vi "SW_Make_Track_overlay.vi"(4 "Pen properties":T1, 5 "Full track array":T2(array[cluster]), 6 "Full trace color":u32(colorbox)=16711680, 7 "Picture in":picture) -> (1 "Picture out":picture)   [LabVIEW 2016]
panel:
  in  "Input colors array":u32[](array[colorbox])=[255, 65535, 6618880, 16776960, 16744448, 16711680]
  out "Colors array":u32[](array[colorbox])
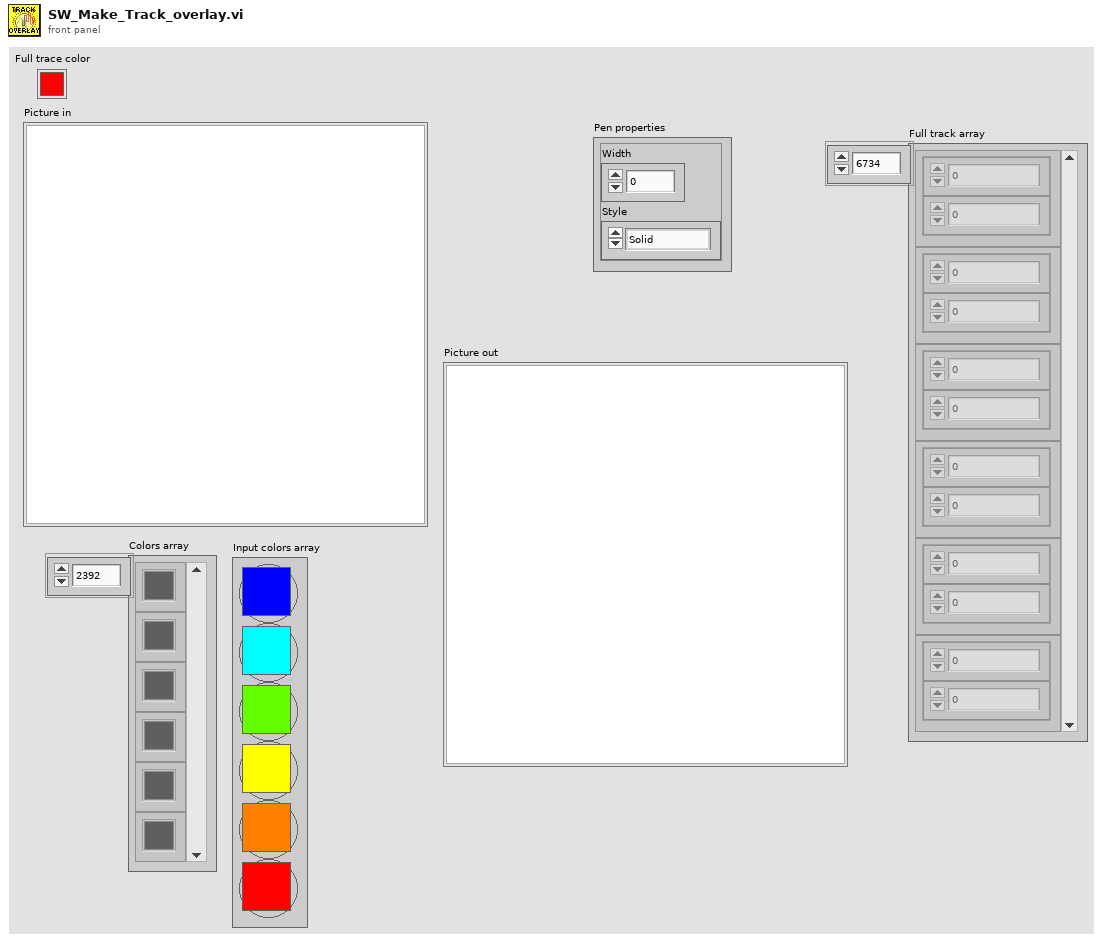
[diagram p1: front panel]
types:
  T1 = cluster{"Width":u16, "Style":enum32{"Solid", "Dash", "Dot", "DashDot", "DashDotDot"}}
  T2 = cluster{"Numeric Control":dbl, "Numeric Control":dbl}[]
  T3 = cluster{"Numeric Control":dbl, "Numeric Control":dbl}
  T4 = cluster{"Numeric Control":i16, "Numeric Control":i16}
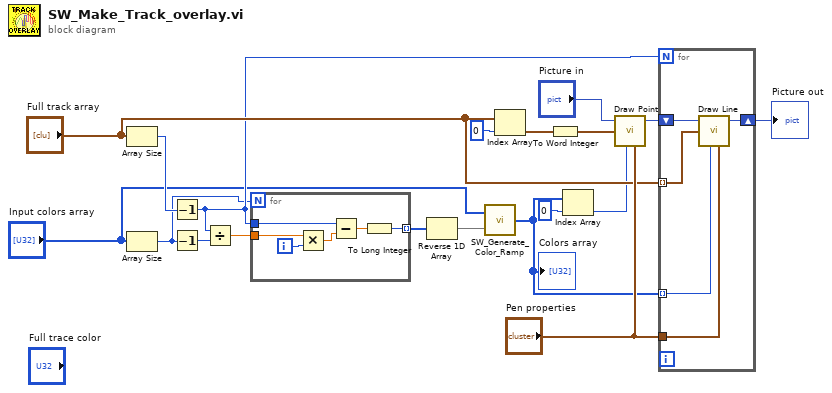
[diagram p0: block diagram]
diagram:
  n1 = Array Size(array="Full track array") -> (size(s)=w11:i32)
  n2 = Array Size(array="Input colors array") -> (size(s)=w4:i32)
  n3 = Decrement(x=w11) -> (x-1=w6:i32)
  n4 = Decrement(x=w4) -> (x-1=w9:i32)
  n5 = Divide(x=w6, y=w9) -> (x/y=w10:dbl)
  n6 = for {
    N: w4 -> [_]
    tunnel: [w20] -> w8 mode=indexing
    tunnel: w6 -> [w25]
    tunnel: w10 -> [w23]
    i -> [w21]
    n7 = Multiply(x=w23, y=w21) -> (x*y=w24:dbl)
    n8 = Subtract(x=w25, y=w24) -> (x-y=w22:dbl)
    n9 = To Long Integer(number=w22) -> (32bit integer=w20:i32)
  }
  n10 = Reverse 1D Array(array=w8) -> (reversed array=w7:i32[])
  n11 = call "SW_Generate_Color_Ramp.vi"("Colors rel. pos."=w7, "Colors array"="Input colors array") -> ("Colors array"=w3:u32[])
  "Colors array" <- w3
  n12 = Index Array(array="Full track array", index=0) -> (element=w15:T3)
  n13 = To Word Integer(number=w15) -> (16bit integer=w13:T4)
  n14 = Index Array(array=w3, index=0) -> (element=w1:u32)
  n15 = call <vilib>:"Draw Point.vi"("picture"="Picture in", "point(x,y)"=w13, "color(black)"=w1, "pen"="Pen properties") -> ("new picture"=w17:picture)  [unwired: 5 in]
  n16 = for {
    N: w6 -> [_]
    tunnel: "Pen properties" -> [w30]
    shift-right: [w29] -> w19
    shift-left: w17 -> [w27]
    tunnel: "Full track array" -> [w28] mode=indexing
    tunnel: w3 -> [w26] mode=indexing
    n17 = call <vilib>:"Draw Line.vi"("picture"=w27, "end point"=w28, "color(black)"=w26, "pen"=w30) -> ("new picture"=w29:picture)  [unwired: 5 in]
  }
  "Picture out" <- w19
